vi "test-trajectory-generate-00.vi"() -> ()   [LabVIEW 2019]
uses:
  <vilib>/Rock Robotics/WPI/ThirdParty/JAS_Junk/TrajLib/TRAJ_STATE.ctl
  <vilib>/Rock Robotics/WPI/ThirdParty/JAS_Junk/TrajLib/POSE2D.ctl
  <vilib>/Rock Robotics/WPI/ThirdParty/JAS_Junk/TrajLib/TRANSLATION2D.ctl
  <vilib>/Rock Robotics/WPI/ThirdParty/JAS_Junk/TrajLib/ROTATION2D.ctl
  <vilib>/Rock Robotics/WPI/ThirdParty/JAS_Junk/TrajLib/Pose_TransformBy.vi
  <vilib>/Rock Robotics/WPI/ThirdParty/JAS_Junk/TrajLib/Util_CalcDist.vi
  <vilib>/Rock Robotics/WPI/ThirdParty/JAS_Junk/TrajLib/Translation_RotateBy.vi
  <vilib>/Rock Robotics/WPI/ThirdParty/JAS_Junk/TrajLib/Translation_Plus.vi
  <vilib>/Rock Robotics/WPI/ThirdParty/JAS_Junk/TrajLib/Rotation_Plus.vi
  <vilib>/Rock Robotics/WPI/ThirdParty/JAS_Junk/TrajLib/Pose_New_TRRO.vi
  <vilib>/Rock Robotics/WPI/ThirdParty/JAS_Junk/TrajLib/Rotation_RotateBy.vi
  <vilib>/Rock Robotics/WPI/ThirdParty/JAS_Junk/TrajLib/Rotation_CreateXY.vi
  <vilib>/Rock Robotics/WPI/ThirdParty/JAS_Junk/TrajLib/Trajectory_Library.lvlib
panel:
  out "Accel\nExceeded (F)":bool
  out "Speed\nExceeded  (F)":bool
  out "TotalTImeSecs":dbl
  out "States":T1[](array[typedef]) {"POSE"."ROTATION"."SIN" format="%13.4f"; "POSE"."ROTATION"."COS" format="%13.4f"; "POSE"."ROTATION"."VALUE" format="%13.4f"; "POSE"."TRANSLATION"."Y" format="%14.3f"; "POSE"."TRANSLATION"."X" format="%14.3f"}
  out "XY Graph":cluster{dbl[], dbl[]}(graph)
  out "Numb\nWaypoints":i32
  out "All Interior \nwayPoints\nFound (True)":bool
  out "end rot = 0":dbl
  out "end y = 0":dbl
  out "end x = 0":dbl
  out "start rot = 0":dbl
  out "start y = 0":dbl
  out "start x = 0":dbl
  out "max dtheta < 0.0872":dbl
  out "max dy < 0.00127":dbl
  out "max dx  < 0.127":dbl
  out "Overall Error":errorcluster
  out "Elements":i32
  out "Elapsed Time":dbl
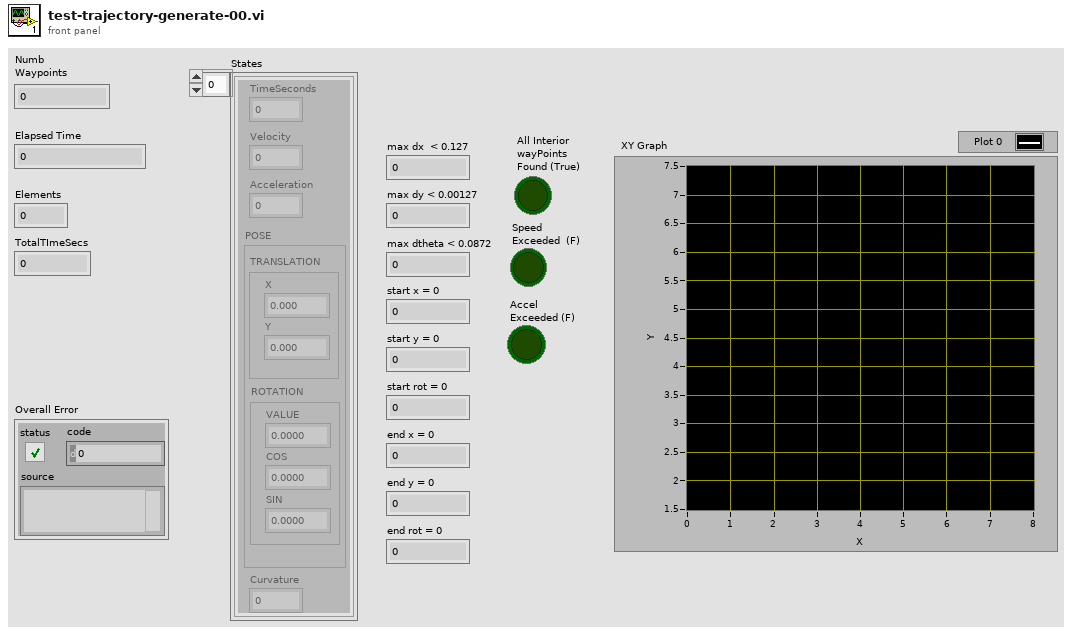
[diagram p1: front panel]
types:
  T1 = typedef "Trajectory_Library.lvlib/TRAJ_STATE.ctl" = cluster{"TimeSeconds":dbl, "Velocity":dbl, "Acceleration":dbl, "POSE":T2, "Curvature":dbl}
  T2 = typedef "Trajectory_Library.lvlib/POSE2D.ctl" = cluster{"TRANSLATION":T3, "ROTATION":T4}
  T3 = typedef "Trajectory_Library.lvlib/TRANSLATION2D.ctl" = cluster{"X":dbl, "Y":dbl}
  T4 = typedef "Trajectory_Library.lvlib/ROTATION2D.ctl" = cluster{"VALUE":dbl, "COS":dbl, "SIN":dbl}
  T5 = typedef "Trajectory_Library.lvlib/TRANSFORM2D.ctl" = cluster{"TRANSLATION":T3, "ROTATION":T4}
  T6 = typedef "Trajectory_Library.lvlib/TRAJ_CONFIG.ctl" = cluster{"MaxVelocity":dbl, "Max Acceleration":dbl, "StartVelocity":dbl, "End Velocity":dbl, "Reversed":bool, "DiffDrKineConstntDefined":bool, "CentAcellConstntDefined":bool, "DiffDrVoltConstntDefined":bool, "DIFF_DRIVE_KINE_CONSTRAINT":T7, "CENTRIPETAL_ACCEL_CONSTRAINT":T9, "SwerveDrKineConstntDefined":bool, "SWERVE_DRIVE_KINE_CONSTRAINT":T10, "DIFF_DRIVE_VOLTAGE_CONSTRAINT":T13, "MECANUM_DRIVE_KINE_CONSTRAINT":T15, "MecanumDrKineConstntDefined":bool}
  T7 = typedef "Trajectory_Library.lvlib/TRAJ_CONSTRAINT_DIIF_DRIVE_KINEMATICS.ctl" = cluster{"Max Speed (M/S)":dbl, "DIFF_DRIVE_KINEMATICS":T8}
  T8 = typedef "Trajectory_Library.lvlib/DIFF_DRIVE_KINEMATICS.ctl" = cluster{"TrackWidth_Meters":dbl}
  T9 = typedef "Trajectory_Library.lvlib/TRAJ_CONSTRAINT_CENTRIPETAL_ACCEL.ctl" = cluster{"Max Cent Accel":dbl}
  T10 = typedef "Trajectory_Library.lvlib/TRAJ_CONSTRAINT_SWERVE_DRIVE_KINEMATICS.ctl" = cluster{"Max Speed (M/S)":dbl, "SwerveKinematics":T11}
  T11 = typedef "Trajectory_Library.lvlib/SWERVE_DRIVE_KINEMATICS.ctl" = cluster{"NumModules":i32, "InverseKinematics":T12, "ForwardKinematics":T12, "Modules":T3[], "PrevCoR":T3}
  T12 = typedef "NI_Matrix.lvlib/RealMatrix.ctl" = dbl[][]
  T13 = typedef "Trajectory_Library.lvlib/TRAJ_CONSTRAINT_DIIF_DRIVE_VOLTAGE.ctl" = cluster{"Max Voltage":dbl, "DIFF_DRIVE_KINEMATICS":T8, "SIMPLE_MOTOR_FF":T14}
  T14 = typedef "Trajectory_Library.lvlib/SIMPLE_MOTOR_FF.ctl" = cluster{"Ks":dbl, "Kv":dbl, "Ka":dbl}
  T15 = typedef "Trajectory_Library.lvlib/TRAJ_CONSTRAINT_MECA_DRIVE_KINEMATICS.ctl" = cluster{"Max Speed (M/S)":dbl, "MECA_DRIVE_KINEMATICS":T16}
  T16 = typedef "Trajectory_Library.lvlib/MECA_DRIVE_KINEMATICS.ctl" = cluster{"FrontLeft":T3, "FrontRight":T3, "RearLeft":T3, "RearRight":T3, "InverseKinematics":T12, "ForwardKinematics":T12, "PrevCoR":T3}
  T17 = typedef "Trajectory_Library.lvlib/TRAJECTORY.ctl" = cluster{"TotalTImeSecs":dbl, "States":T1[]}
  T18 = typedef "Trajectory_Library.lvlib/TWIST2D.ctl" = cluster{"dX":dbl, "dY":dbl, "dTHETA":dbl}
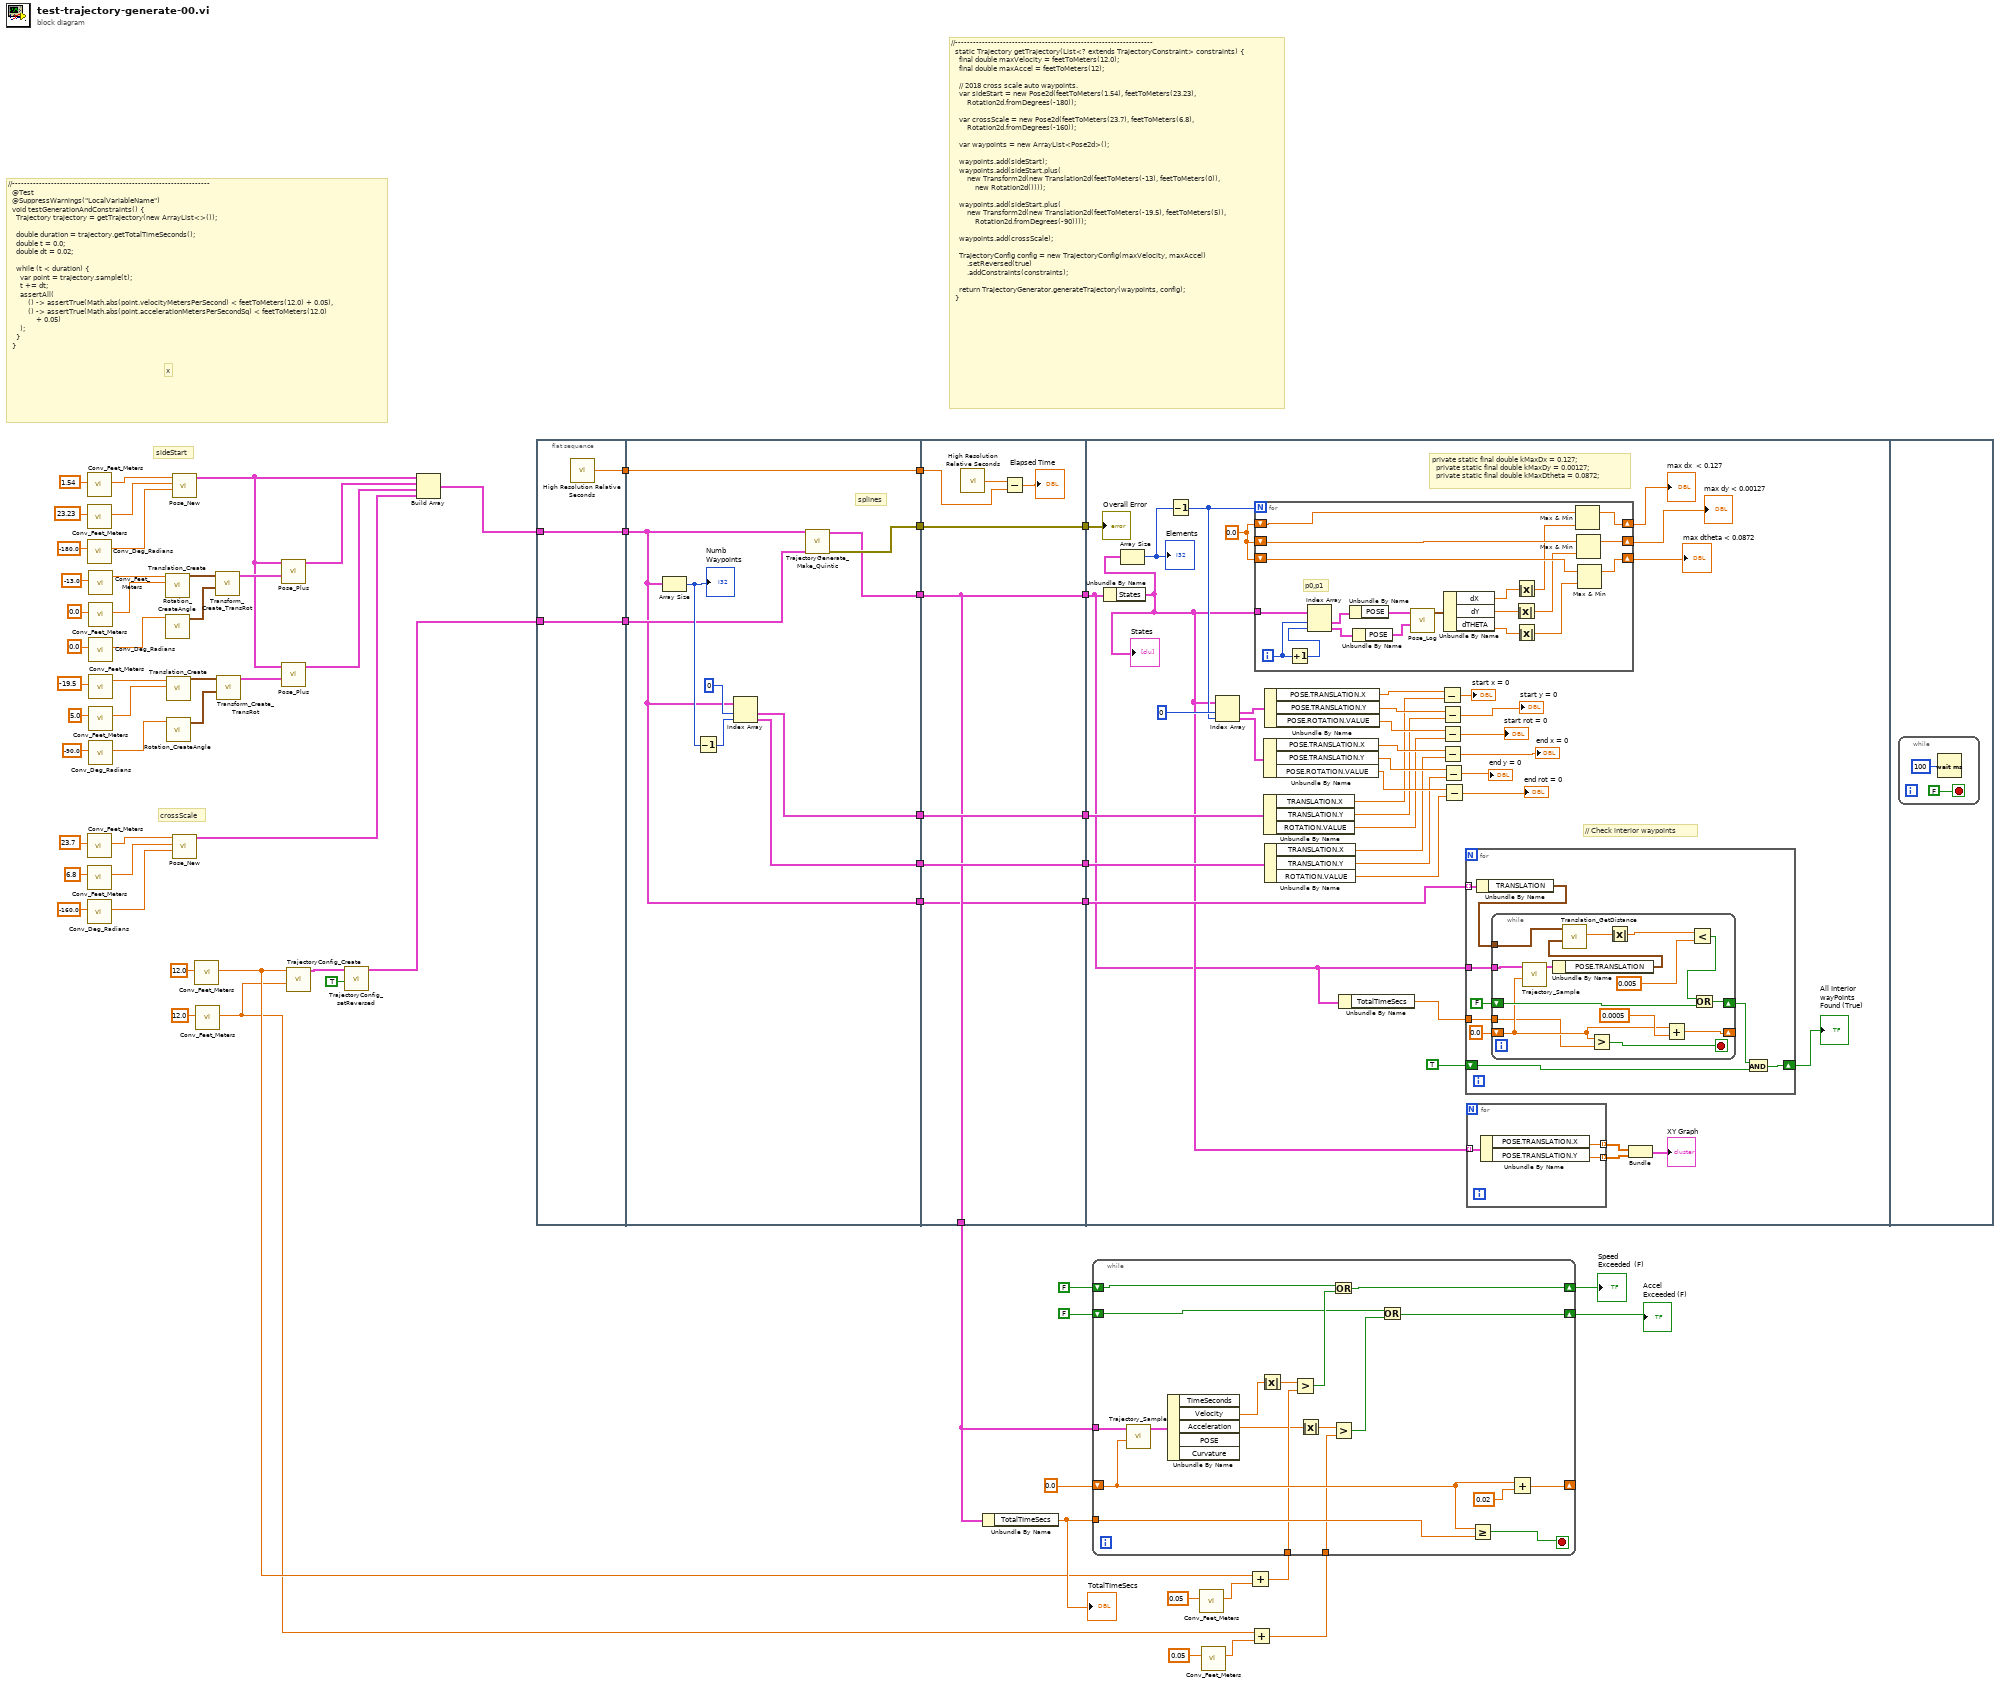
[diagram p0: block diagram]
diagram:
  # "//------------------------------------------------------------------\n  @Test\n  @SuppressWarnings(\"LocalVariableName\")\n  void testGenerationAndConstraints() {\n    Trajectory trajectory = getTrajectory(new ArrayList<>());\n\n    double duration = trajectory.getTotalTimeSeconds();\n    double t = 0.0;\n    double dt = 0.02;\n\n    while (t < duration) {\n      var point = trajectory.sample(t);\n      t += dt;\n      assertAll(\n          () -> assertTrue(Math.abs(point.velocityMetersPerSecond) < feetToMeters(12.0) + 0.05),\n          () -> assertTrue(Math.abs(point.accelerationMetersPerSecondSq) < feetToMeters(12.0)\n              + 0.05)\n      );\n    }\n  }"
  # "crossScale"
  # "sideStart"
  # "//------------------------------------------------------------------\n  static Trajectory getTrajectory(List<? extends TrajectoryConstraint> constraints) {\n    final double maxVelocity = feetToMeters(12.0);\n    final double maxAccel = feetToMeters(12);\n\n    // 2018 cross scale auto waypoints.\n    var sideStart = new Pose2d(feetToMeters(1.54), feetToMeters(23.23),\n        Rotation2d.fromDegrees(-180));\n\n    var crossScale = new Pose2d(feetToMeters(23.7), feetToMeters(6.8),\n        Rotation2d.fromDegrees(-160));\n\n    var waypoints = new ArrayList<Pose2d>();\n\n    waypoints.add(sideStart);\n    waypoints.add(sideStart.plus(\n        new Transform2d(new Translation2d(feetToMeters(-13), feetToMeters(0)),\n            new Rotation2d())));\n\n    waypoints.add(sideStart.plus(\n        new Transform2d(new Translation2d(feetToMeters(-19.5), feetToMeters(5)),\n            Rotation2d.fromDegrees(-90))));\n\n    waypoints.add(crossScale);\n\n    TrajectoryConfig config = new TrajectoryConfig(maxVelocity, maxAccel)\n        .setReversed(true)\n        .addConstraints(constraints);\n\n    return TrajectoryGenerator.generateTrajectory(waypoints, config);\n  }"
  # "x"
  n1 = call <vilib>:"Conv_Feet_Meters.vi"("Feet"=1.54) -> ("Meters"=w59:dbl)  [unwired: 10 in]
  n2 = call <vilib>:"Conv_Feet_Meters.vi"("Feet"=23.23) -> ("Meters"=w58:dbl)  [unwired: 10 in]
  n3 = call <vilib>:"Conv_Deg_Radians.vi"("Degress"=-180.0) -> ("Radians"=w57:dbl)  [unwired: 10 in]
  n4 = call <vilib>:"Conv_Feet_Meters.vi"("Feet"=23.7) -> ("Meters"=w53:dbl)  [unwired: 10 in]
  n5 = call <vilib>:"Conv_Feet_Meters.vi"("Feet"=6.8) -> ("Meters"=w52:dbl)  [unwired: 10 in]
  n6 = call <vilib>:"Conv_Deg_Radians.vi"("Degress"=-160.0) -> ("Radians"=w51:dbl)  [unwired: 10 in]
  n7 = call <vilib>:"Conv_Feet_Meters.vi"("Feet"=-13.0) -> ("Meters"=w46:dbl)  [unwired: 10 in]
  n8 = call <vilib>:"Conv_Feet_Meters.vi"("Feet"=0.0) -> ("Meters"=w45:dbl)  [unwired: 10 in]
  n9 = call <vilib>:"Conv_Deg_Radians.vi"("Degress"=0.0) -> ("Radians"=w44:dbl)  [unwired: 10 in]
  n10 = call <vilib>:"Conv_Feet_Meters.vi"("Feet"=-19.5) -> ("Meters"=w37:dbl)  [unwired: 10 in]
  n11 = call <vilib>:"Conv_Feet_Meters.vi"("Feet"=5.0) -> ("Meters"=w36:dbl)  [unwired: 10 in]
  n12 = call <vilib>:"Conv_Deg_Radians.vi"("Degress"=-90.0) -> ("Radians"=w35:dbl)  [unwired: 10 in]
  n13 = call <vilib>:"Translation_Create.vi"("Y"=w45, "X"=w46) -> ("TRANSLATION"=w43:T3)  [unwired: 9 in]
  n14 = call <vilib>:"Rotation_CreateAngle.vi"("Angle"=w44) -> ("ROTATION"=w42:T4)  [unwired: 10 in]
  n15 = call <vilib>:"Translation_Create.vi"("Y"=w36, "X"=w37) -> ("TRANSLATION"=w34:T3)  [unwired: 9 in]
  n16 = call <vilib>:"Rotation_CreateAngle.vi"("Angle"=w35) -> ("ROTATION"=w33:T4)  [unwired: 10 in]
  n17 = call <vilib>:"Pose_New.vi"("Heading"=w57, "Y"=w58, "X"=w59) -> ("out POSe"=w32:T2)  [unwired: 8 in]
  n18 = call <vilib>:"Pose_New.vi"("Heading"=w51, "Y"=w52, "X"=w53) -> ("out POSe"=w29:T2)  [unwired: 8 in]
  n19 = call <vilib>:"Conv_Feet_Meters.vi"("Feet"=12.0) -> ("Meters"=w13:dbl)  [unwired: 10 in]
  n20 = call <vilib>:"Conv_Feet_Meters.vi"("Feet"=12.0) -> ("Meters"=w3:dbl)  [unwired: 10 in]
  n21 = call <vilib>:"Transform_Create_TransRot.vi"("ROTATION"=w42, "TRANSLATION"=w43) -> ("TRANSFORM"=w50:T5)  [unwired: 9 in]
  n22 = call <vilib>:"Transform_Create_TransRot.vi"("ROTATION"=w33, "TRANSLATION"=w34) -> ("TRANSFORM"=w41:T5)  [unwired: 9 in]
  n23 = call <vilib>:"Pose_Plus.vi"("other TRANSFORM"=w50, "in POSE"=w32) -> ("out POSE"=w31:T2)  [unwired: 9 in]
  n24 = call <vilib>:"Pose_Plus.vi"("other TRANSFORM"=w41, "in POSE"=w32) -> ("out POSE"=w30:T2)  [unwired: 9 in]
  n25 = call <vilib>:"TrajectoryConfig_Create.vi"("MaxAcceleration"=w3, "MaxVelocity"=w13) -> ("TRAJECTORY_CONFIG"=w25:T6)  [unwired: 9 in]
  n26 = call <vilib>:"TrajectoryConfig_setReversed.vi"("Reversed"=TRUE, "inTRAJECTORY_CONFIG"=w25) -> ("outTRAJECTORY_CONFIG"=w21:T6)  [unwired: 9 in]
  n27 = Build Array(w32, w31, w30, w29) -> (w23:T2[])
  n28 = flat-sequence {
    tunnel: [w72] -> w69
    tunnel: [w71] -> w24
    tunnel: w23 -> [w71]
    tunnel: [w70] -> w22
    tunnel: w21 -> [w70]
    tunnel: [w82] -> w68
    tunnel: w69 -> [w82]
    tunnel: [w78] -> w66
    tunnel: [w77] -> w64
    tunnel: w24 -> [w73]
    tunnel: w22 -> [w74]
    tunnel: [w76] -> w20
    tunnel: [w75] -> w19
    tunnel: [w73] -> w1
    tunnel: w68 -> [w90]
    tunnel: [w85] -> w67
    tunnel: w66 -> [w87]
    tunnel: [w87] -> w65
    tunnel: w64 -> [w86]
    tunnel: [w86] -> w63
    tunnel: w20 -> [w85]
    tunnel: w19 -> [w84]
    tunnel: [w84] -> w18
    tunnel: [w84] -> w15
    tunnel: [w83] -> w2
    tunnel: w1 -> [w83]
    tunnel: w67 -> [w129]
    tunnel: w65 -> [w123]
    tunnel: w63 -> [w122]
    tunnel: w18 -> [w91]
    tunnel: w2 -> [w94]
    frame #0 {
      n29 = call <vilib>:"High Resolution Relative Seconds.vi"() -> ("relative seconds"=w72:dbl)
    }
    frame #1 {
      # "splines"
      n30 = Array Size(array=w73) -> (size(s)=w79:i32)
      "Numb\nWaypoints" <- w79
      n31 = Decrement(x=w79) -> (x-1=w80:i32)
      n32 = Index Array(array=w73, index #1=0 ("index"), index #2=w80) -> (element #1=w78:T2, element #2=w77:T2)
      n33 = call <vilib>:"TrajectoryGenerate_Make_Quintic.vi"("traj_config"=w74, "waypointPOSE"=w73) -> ("error out"=w76:errorcluster, "TRAJECTORY"=w75:T17)  [unwired: 8 in]
    }
    frame #2 {
      n34 = call <vilib>:"High Resolution Relative Seconds.vi"() -> ("relative seconds"=w88:dbl)
      n35 = Subtract(x=w88, y=w90) -> (x-y=→"Elapsed Time":dbl)
    }
    frame #3 {
      w127 = 0.0
      # "// Check interior waypoints"
      # "private static final double kMaxDx = 0.127;\n  private static final double kMaxDy = 0.00127;\n  private static final double kMaxDtheta = 0.0872;"
      n36 = Unbundle By Name(w91) -> ("States"=w92:T1[])
      "States" <- w92
      n37 = Array Size(array=w92) -> (size(s)=w128:i32)
      "Elements" <- w128
      n38 = Decrement(x=w128) -> (x-1=w120:i32)
      n39 = Index Array(array=w92, index #1=0 ("index"), index #2=w120) -> (element #1=w119:T1, element #2=w118:T1)
      n40 = for {
        N: w120 -> [_]
        tunnel: w92 -> [w174]
        shift-right: [w165] -> w126
        shift-left: w127 -> [w162]
        shift-right: [w163] -> w124
        shift-left: w127 -> [w160]
        shift-right: [w164] -> w125
        shift-left: w127 -> [w161]
        i -> [w176]
        # "p0,p1"
        n41 = Increment(x=w176) -> (x+1=w175:i32)
        n42 = Index Array(array=w174, index #1=w176, index #2=w175) -> (element #1=w173:T1, element #2=w172:T1)
        n43 = Unbundle By Name(w173) -> ("POSE"=w171:T2)
        n44 = Unbundle By Name(w172) -> ("POSE"=w170:T2)
        n45 = call <vilib>:"Pose_Log.vi"("end POSE"=w170, "in POSE"=w171) -> ("out TWIST"=w169:T18)  [unwired: 9 in]
        n46 = Unbundle By Name(w169) -> ("dX"=w166:dbl, "dY"=w167:dbl, "dTHETA"=w168:dbl)
        n47 = Absolute Value(x=w167) -> (abs(x)=w158:dbl)
        n48 = Absolute Value(x=w166) -> (abs(x)=w159:dbl)
        n49 = Absolute Value(x=w168) -> (abs(x)=w157:dbl)
        n50 = Max & Min(x=w162, y=w159) -> (max(x,y)=w165:dbl)  [unwired: 1 out]
        n51 = Max & Min(x=w161, y=w158) -> (max(x,y)=w164:dbl)  [unwired: 1 out]
        n52 = Max & Min(x=w160, y=w157) -> (max(x,y)=w163:dbl)  [unwired: 1 out]
      }
      "max dx  < 0.127" <- w126
      "max dy < 0.00127" <- w125
      "max dtheta < 0.0872" <- w124
      n53 = Unbundle By Name(w118) -> ("POSE.TRANSLATION.X"=w114:dbl, "POSE.TRANSLATION.Y"=w113:dbl, "POSE.ROTATION.VALUE"=w112:dbl)
      n54 = Unbundle By Name(w123) -> ("TRANSLATION.X"=w111:dbl, "TRANSLATION.Y"=w110:dbl, "ROTATION.VALUE"=w109:dbl)
      n55 = Unbundle By Name(w119) -> ("POSE.TRANSLATION.X"=w117:dbl, "POSE.TRANSLATION.Y"=w116:dbl, "POSE.ROTATION.VALUE"=w115:dbl)
      n56 = Unbundle By Name(w122) -> ("TRANSLATION.X"=w108:dbl, "TRANSLATION.Y"=w107:dbl, "ROTATION.VALUE"=w106:dbl)
      n57 = Unbundle By Name(w91) -> ("TotalTImeSecs"=w93:dbl)
      n58 = Subtract(x=w117, y=w111) -> (x-y=→"start x = 0":dbl)
      n59 = Subtract(x=w116, y=w110) -> (x-y=→"start y = 0":dbl)
      n60 = Subtract(x=w115, y=w109) -> (x-y=→"start rot = 0":dbl)
      n61 = Subtract(x=w114, y=w108) -> (x-y=→"end x = 0":dbl)
      n62 = Subtract(x=w113, y=w107) -> (x-y=→"end y = 0":dbl)
      n63 = Subtract(x=w112, y=w106) -> (x-y=→"end rot = 0":dbl)
      n64 = for {
        tunnel: w91 -> [w138]
        shift-right: [w137] -> w98
        shift-left: TRUE -> [w136]
        tunnel: w94 -> [w132] mode=indexing
        tunnel: w93 -> [w130]
        n65 = Unbundle By Name(w132) -> ("TRANSLATION"=w133:T3)
        n66 = while {
          tunnel: w138 -> [w147]
          shift-right: [w153] -> w134
          shift-left: FALSE -> [w152]
          tunnel: w133 -> [w151]
          shift-right: [w149] -> _
          shift-left: 0.0 -> [w141]
          tunnel: w130 -> [w140]
          stop <- w139 stop-if-true
          n67 = call <vilib>:"Trajectory_Sample.vi"("Time"=w141, "InputTRAJECTORY"=w147) -> ("OutputTRAJ_STATE"=w146:T1)  [unwired: 9 in]
          n68 = Unbundle By Name(w146) -> ("POSE.TRANSLATION"=w150:T3)
          n69 = call <vilib>:"Translation_GetDistance.vi"("other Translation"=w150, "In Translation"=w151) -> ("Distance"=w145:dbl)  [unwired: 9 in]
          n70 = Greater?(x=w141, y=w140) -> (0:w139:bool)
          n71 = Absolute Value(x=w145) -> (abs(x)=w144:dbl)
          n72 = Add(x=w141, y=0.0005) -> (x+y=w149:dbl)
          n73 = Less?(x=w144, y=0.005) -> (x < y?=w142:bool)
          n74 = Or(x=w142, y=w152) -> (x .or. y?=w153:bool)
        }
        n75 = And(x=w134, y=w136) -> (x .and. y?=w137:bool)
      }
      "All Interior \nwayPoints\nFound (True)" <- w98
      n76 = for {
        tunnel: [w156] -> w97 mode=indexing
        tunnel: [w155] -> w96 mode=indexing
        tunnel: w92 -> [w154] mode=indexing
        n77 = Unbundle By Name(w154) -> ("POSE.TRANSLATION.X"=w156:dbl, "POSE.TRANSLATION.Y"=w155:dbl)
      }
      n78 = Bundle(w97, w96) -> (→"XY Graph":cluster{dbl[], dbl[]})  [unwired: 1 in]
      "Overall Error" <- w129
    }
    frame #4 {
      n79 = while {
        stop <- FALSE stop-if-true
        n80 = Wait (ms)(milliseconds to wait=u32 100) -> ()  [unwired: 1 out]
      }
    }
  }
  n81 = Unbundle By Name(w15) -> ("TotalTImeSecs"=w16:dbl)
  "TotalTImeSecs" <- w16
  n82 = call <vilib>:"Conv_Feet_Meters.vi"("Feet"=0.05 ("y")) -> ("Meters"=w11:dbl)  [unwired: 10 in]
  n83 = call <vilib>:"Conv_Feet_Meters.vi"("Feet"=0.05 ("y")) -> ("Meters"=w8:dbl)  [unwired: 10 in]
  n84 = Add(x=w13, y=w11) -> (x+y=w10:dbl)
  n85 = Add(x=w3, y=w8) -> (x+y=w6:dbl)
  n86 = while {
    shift-right: [w196] -> _
    shift-left: 0.0 -> [w193]
    tunnel: w16 -> [w194]
    tunnel: w15 -> [w192]
    shift-right: [w188] -> w5
    shift-left: FALSE -> [w186]
    tunnel: w10 -> [w185]
    shift-right: [w181] -> w4
    shift-left: FALSE -> [w179]
    tunnel: w6 -> [w182]
    stop <- w195 stop-if-true
    n87 = call <vilib>:"Trajectory_Sample.vi"("Time"=w193, "InputTRAJECTORY"=w192) -> ("OutputTRAJ_STATE"=w191:T1)  [unwired: 9 in]
    n88 = Unbundle By Name(w191) -> ("Velocity"=w190:dbl, "Acceleration"=w183:dbl)  [unwired: 3 out]
    n89 = Absolute Value(x=w190) -> (abs(x)=w189:dbl)
    n90 = Greater?(x=w189, y=w185) -> (0:w187:bool)
    n91 = Absolute Value(x=w183) -> (abs(x)=w184:dbl)
    n92 = Or(x=w186, y=w187) -> (x .or. y?=w188:bool)
    n93 = Greater?(x=w184, y=w182) -> (0:w180:bool)
    n94 = Or(x=w179, y=w180) -> (x .or. y?=w181:bool)
    n95 = Greater Or Equal?(x=w193, y=w194) -> (x >= y?=w195:bool)
    n96 = Add(x=w193, y=0.02) -> (x+y=w196:dbl)
  }
  "Speed\nExceeded  (F)" <- w5
  "Accel\nExceeded (F)" <- w4
